vi "date & time path generator.vi"(0 "system directory type":T1=2 items=["User Home"=0, "User Desktop"=1, "User Documents"=2, "User Application Data"=3, "User Preferences"=4, "User Temporary"=5, "Public Documents"=6, "Public Application Data"=7, "Public Preferences"=8, "Public Cache"=13, "System Core Libraries"=9, "System Installed Libraries"=10, "Application Files"=11, "Boot Volume Root"=12], 1 "nome da pasta":string, 3 "nome do arquivo":string) -> (8 "path":path)   [LabVIEW 2019]
uses:
  <vilib>/Utility/sysdir.llb/System Directory Type.ctl
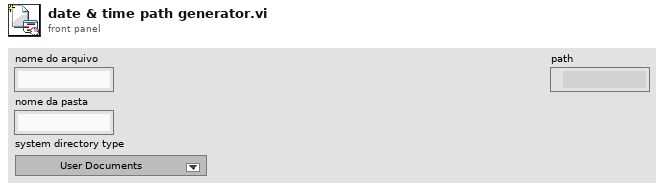
[diagram p1: front panel]
types:
  T1 = typedef "System Directory Type.ctl" = i32
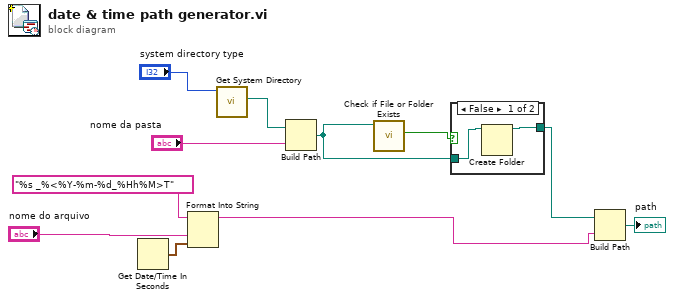
[diagram p0: block diagram]
diagram:
  n1 = Get Date/Time In Seconds() -> (seconds since 1Jan1904=w9:timestamp)
  n2 = Format Into String(format string="%s _%<%Y-%m-%d_%Hh%M>T", "nome do arquivo", w9) -> (resulting string=w2:string)  [unwired: 2 in, 1 out]
  n3 = call <vilib>:"Get System Directory.vi"("system directory type"="system directory type") -> ("system directory"=w6:path)  [unwired: 10 in]
  n4 = Build Path(base path=w6, name or relative path="nome da pasta") -> (appended path=w4:path)
  n5 = call <vilib>:"Check if File or Folder Exists.vi"("path"=w4) -> ("file or folder exists?"=w5:bool)  [unwired: 8 in, 2 out]
  n6 = case shown="False" w5 {
    tunnel: w4 -> [w12 w14]
    tunnel: [w13 w14] -> w3
    frame False {
      n7 = Create Folder(path (use dialog)=w12) -> (created path=w13:path)  [unwired: 2 in, 2 out]
    }
    frame True {
    }
  }
  n8 = Build Path(base path=w3, name or relative path=w2) -> (appended path=→"path":path)
